vi "Begin.vi"() -> (0 "error out":errorcluster)   [LabVIEW 2013]
doc: "Called before other user functions, this VI is expected to open initial I/O refnums, load in file data, and do all program initialization. Notice that the <B>error out</B> terminal is simply used for data flow. Wiring it to other structures or subVIs ensures that this VI runs first."
uses:
  <vilib>/Rock Robotics/WPI/SafetyOutput/WPI_SafetyOutputConfigMenu.ctl
  <vilib>/Rock Robotics/WPI/DriverStation/WPI_DriverStationRobotMode2.ctl
  <vilib>/Rock Robotics/WPI/Joystick/WPI_JoystickDeviceEnum.ctl
  <vilib>/Rock Robotics/SystemInterfaces/DIO/FPGA_DIOChannel.ctl
  <vilib>/Rock Robotics/WPI/Solenoid/WPI_SolenoidChannel.ctl
  <vilib>/Rock Robotics/SystemInterfaces/DIO/FPGA_DIORelayChannel.ctl
  <vilib>/Rock Robotics/SystemInterfaces/AI/FPGA_AIChannel.ctl
  Robot Global Data.vi
  <vilib>/Rock Robotics/WPI/Counter/WPI_CounterDigitalInputToDigitalSource.vi
  <vilib>/Rock Robotics/WPI/Solenoid/WPI_SolenoidOpenSingle.vi
  <vilib>/Rock Robotics/WPI/RobotDrive/WPI_RobotDriveOpen4MotorWithCANJaguar.vi
  <vilib>/Rock Robotics/WPI/Solenoid/WPI_SolenoidOpenDouble.vi
  <vilib>/Rock Robotics/WPI/MotorControl/WPI_MotorControlOpenCANJaguar.vi
  <vilib>/Rock Robotics/WPI/Compressor/WPI_CompressorGetSetRefNum.vi
panel:
  out "error out 2":errorcluster
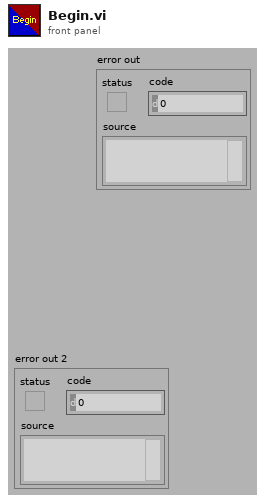
[diagram p1: front panel]
types:
  T1 = typedef "FPGA_DIOChannel.ctl" = enum8{"DIO 1", "DIO 2", "DIO 3", "DIO 4", "DIO 5", "DIO 6", "DIO 7", "DIO 8", "DIO 9", "DIO 10", "DIO 11", "DIO 12", "DIO 13", "DIO 14", "Invalid"}
  T2 = typedef "FPGA_DIORelayChannel.ctl" = enum8{"Relay 1", "Relay 2", "Relay 3", "Relay 4", "Relay 5", "Relay 6", "Relay 7", "Relay 8", "Invalid"}
  T3 = typedef "FPGA_AIChannel.ctl" = enum8{"AI 1", "AI 2", "AI 3", "AI 4", "AI 5", "AI 6", "AI 7", "AI 8", "Invalid"}
  T4 = typedef "WPI_SolenoidChannel.ctl" = enum8{"Solenoid 1", "Solenoid 2", "Solenoid 3", "Solenoid 4", "Solenoid 5", "Solenoid 6", "Solenoid 7", "Solenoid 8", "Invalid"}
  T5 = typedef "WPI_JoystickDeviceEnum.ctl" = enum16{"USB 1", "USB 2", "USB 3", "USB 4", "Kinect 1", "Kinect 2"}
  T6 = typedef "WPI_DriverStationRobotMode2.ctl" = enum16{"Autonomous Disabled", "Autonomous Enabled", "Teleop Disabled", "Teleop Enabled", "Timeout", "Finish", "Test Disabled", "Test Enabled"}
  T7 = typedef "WPI_SafetyOutputConfigMenu.ctl" = enum16{"Enable", "Disable"}
  T8 = typedef "WPI_DigitalInputDevRef.ctl" = cluster{"DevStatus":errorcluster, "DIO Channel":T1, "Digital Module":T9}
  T9 = typedef "FPGA_TypedefDigitalModule.ctl" = enum16{"Digital Module 1", "Digital Module 2"}
  T10 = typedef "FPGA_CounterEncoderSourceConvertionLVSourceType.ctl" = cluster{"DevStatus":errorcluster, "AnalogTriggerMode?":bool, "DigitalMode":cluster{"Digital Module":T9, "DIO Channel":T11}, "AnalogTriggerMode":cluster{"AnalogTriggerIndex":T12, "OutputType":T13}}
  T11 = typedef "FPGA_DIODigitalSourceChannel.ctl" = enum8{"DIO 1", "DIO 2", "DIO 3", "DIO 4", "DIO 5", "DIO 6", "DIO 7", "DIO 8", "DIO 9", "DIO 10", "DIO 11", "DIO 12", "DIO 13", "DIO 14", "Disabled"}
  T12 = typedef "FPGA_AnalogTriggerIndex.ctl" = enum8{"Trig 0", "Trig 1", "Trig 2", "Trig 3", "Trig 4", "Trig 5", "Trig 6", "Trig 7", "Invalid"}
  T13 = typedef "FPGA_AnalogTriggerOutType.ctl" = enum16{"InWindow", "TriggerState", "Rising", "Falling"}
  T14 = typedef "WPI_JoystickDevRef.ctl" = cluster{"Device":T5}
  T15 = typedef "WPI_RobotDriveDevRef.ctl" = cluster{"DevStatus":errorcluster, "Motors[]":T16[], "Square Inputs":bool, "Max Output":dbl, "Isochronous":bool}
  T16 = typedef "WPI_MotorControlDeviceRef.ctl" = cluster{"DeviceStatus":errorcluster, "Type":enum16{"PWM", "CAN"}, "PWM":cluster{"Digital Module":T9, "PWM Channel":T17, "DeadBand":T18}, "CAN":cluster{"Device Number":u8, "Control Mode":T19, "Semaphore":T20, "Max Vout":dbl}, "Invert":bool, "TransformRef":T21, "InvTransformRef":T21}
  T17 = typedef "FPGA_DIOPWMChannel.ctl" = enum8{"PWM 1", "PWM 2", "PWM 3", "PWM 4", "PWM 5", "PWM 6", "PWM 7", "PWM 8", "PWM 9", "PWM 10", "Invalid"}
  T18 = typedef "WPI_PWMDeadband.ctl" = cluster{"Name":string, "maxPositivePwm":i32, "minPositivePwm":i32, "centerPwm":i32, "maxNegativePwm":i32, "minNegativePwm":i32, "angularRange":u16}
  T19 = typedef "WPI_CANJaguar_ControlMode.ctl" = enum8{"Percent VBus", "Current", "Speed", "Position", "Voltage"}
  T20 = typedef "Semaphore RefNum" = refnum<k1>
  T21 = typedef "WPI_PWMTransform_ConPane.ctl" = refnum<vi>
  T22 = typedef "WPI_EncoderDevRef.ctl" = cluster{"DevStatus":errorcluster, "EncoderIndex":T23, "CounterIndex":T24, "DistancePerCount":dbl, "Decoding Type":T25}
  T23 = typedef "FPGA_EncoderIdx.ctl" = enum8{"Enc 0", "Enc 1", "Enc 2", "Enc 3", "Invalid"}
  T24 = typedef "FPGA_CounterCtrSystemIndex.ctl" = enum8{"Ctr 0", "Ctr 1", "Ctr 2", "Ctr 3", "Ctr 4", "Ctr 5", "Ctr 6", "Ctr 7", "Invalid"}
  T25 = typedef "WPI_EncoderType.ctl" = enum16{"1x", "2x", "4x"}
  T26 = typedef "WPI_AnalogChannelDevRef.ctl" = cluster{"DevStatus":errorcluster, "Analog Module":T27, "Analog Channel":T3}
  T27 = typedef "FPGA_TypedefAnalogModule.ctl" = enum16{"Analog Module 1", "Analog Module 2"}
  T28 = typedef "WPI_CompressorDevRef.ctl" = cluster{"DevStatus":errorcluster, "DigitalInputDevRef":T8, "RelayDevRef":T29}
  T29 = typedef "WPI_RelayDevRef.ctl" = cluster{"DevStatus":errorcluster, "Relay Channel":T2, "Digital Module":T9, "Relay Direction":T30}
  T30 = typedef "WPI_RelayDirection.ctl" = enum16{"Both directions", "Forward only", "Reverse only"}
  T31 = typedef "WPI_SolenoidDevRef.ctl" = cluster{"DevStatus":errorcluster, "Solenoid Module":T32, "Forward Solenoid Channel":T4, "Reverse Solenoid Channel":T4}
  T32 = typedef "FPGA_TypedefSolenoidModule.ctl" = enum16{"Solenoid Module 1", "Solenoid Module 2"}
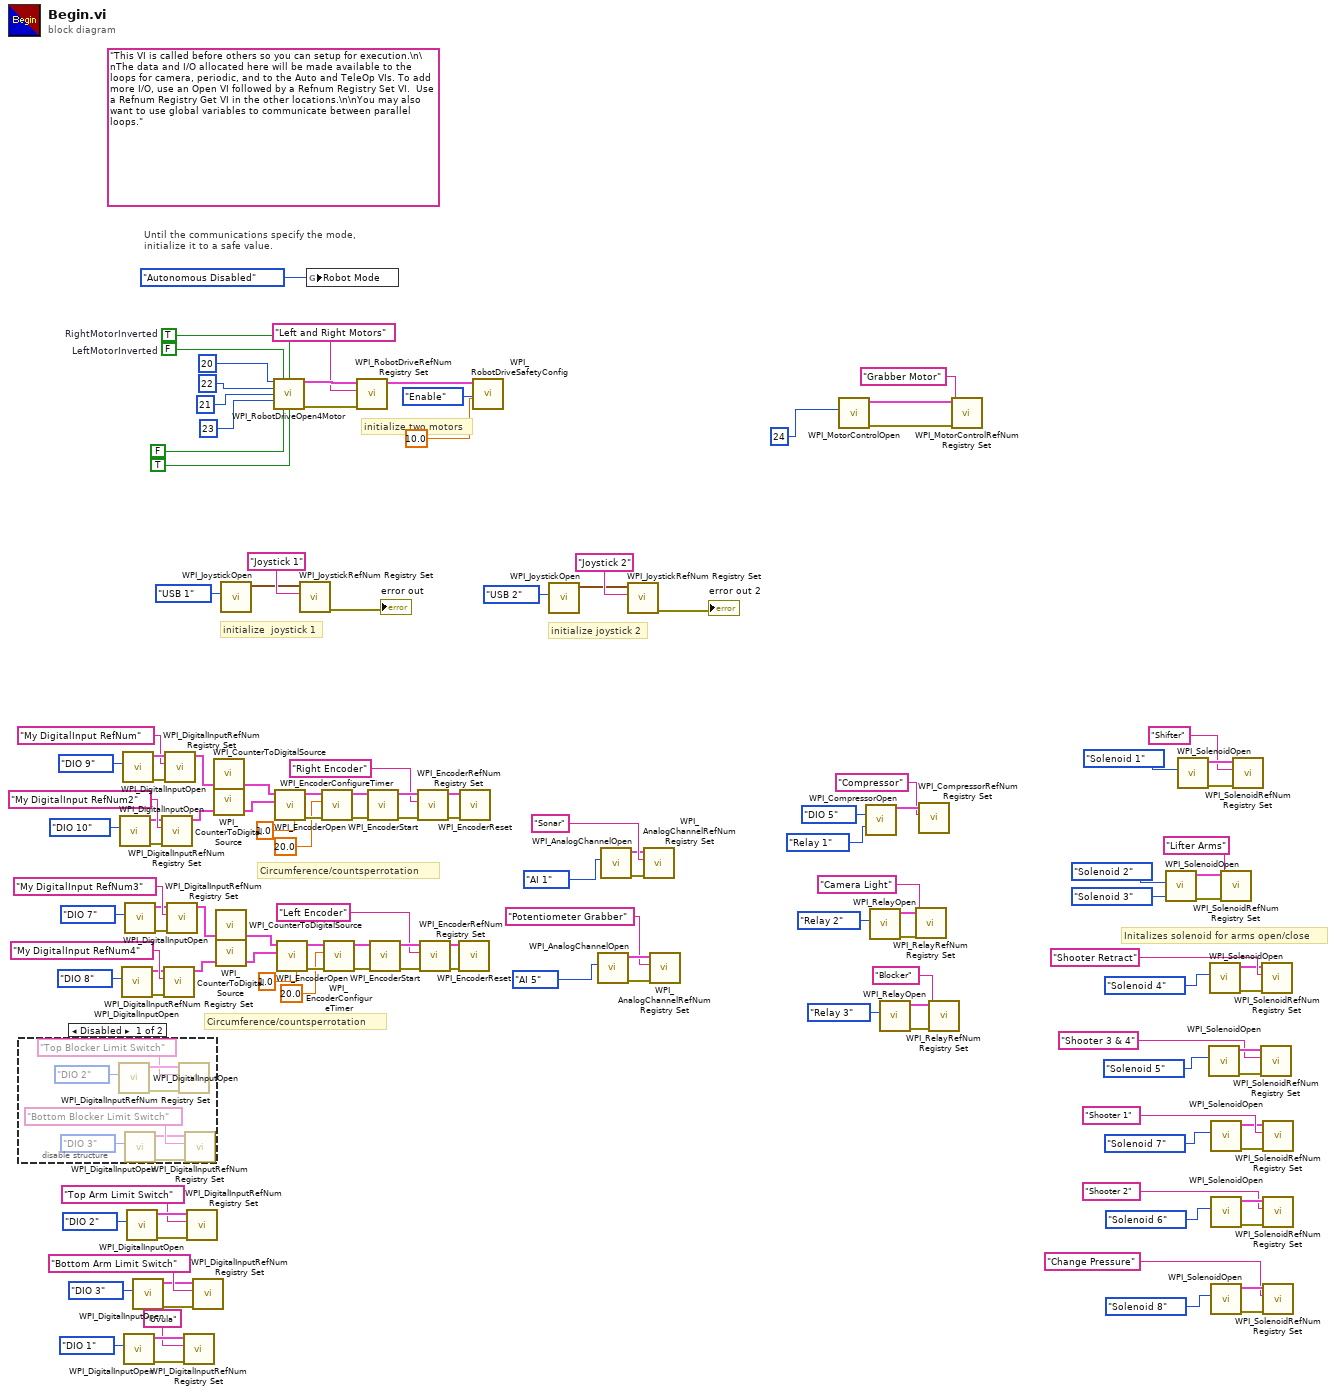
[diagram p0: block diagram]
diagram:
  (unwired) "This VI is called before others so you can setup for execution.\n\nThe data and I/O allocated here will be made available to the loops for camera, periodic, and to the Auto and TeleOp VIs. To add more I/O, use an Open VI followed by a Refnum Registry Set VI.  Use a Refnum Registry Get VI in the other locations.\n\nYou may also want to use global variables to communicate between parallel loops."
  w77 = FALSE  # LeftMotorInverted
  w76 = TRUE  # RightMotorInverted
  # "Initalizes solenoid for arms open/close"
  # "initialize joystick 2"
  # "Circumference/countsperrotation"
  # "Circumference/countsperrotation"
  # "initialize  joystick 1"
  # "Until the communications specify the mode,\ninitialize it to a safe value."
  # "initialize two motors"
  n1 = disable-structure shown="Disabled" {
    frame Disabled {
      n2 = call <vilib>:"WPI_DigitalInputOpen.vi"("DIO Channel"=FPGA_DIOChannel."DIO 2") -> ("error out"=w142:errorcluster, "DigitalInputDevRef"=w141:T8)  [unwired: 9 in]
      n3 = call <vilib>:"WPI_DigitalInputOpen.vi"("DIO Channel"=FPGA_DIOChannel."DIO 3") -> ("error out"=w135:errorcluster, "DigitalInputDevRef"=w136:T8)  [unwired: 9 in]
      n4 = call <vilib>:"WPI_DigitalInputRefNum Registry Set.vi"("error in (no error)"=w142, "refnum name"="Top Blocker Limit Switch", "DigitalInputDevRef"=w141) -> ()  [unwired: 7 in, 2 out]
      n5 = call <vilib>:"WPI_DigitalInputRefNum Registry Set.vi"("error in (no error)"=w135, "refnum name"="Bottom Blocker Limit Switch", "DigitalInputDevRef"=w136) -> ()  [unwired: 7 in, 2 out]
    }
    frame Enabled {
    }
  }
  n6 = call <vilib>:"WPI_DigitalInputOpen.vi"("DIO Channel"=FPGA_DIOChannel."DIO 10") -> ("error out"=w106:errorcluster, "DigitalInputDevRef"=w107:T8)  [unwired: 9 in]
  n7 = call <vilib>:"WPI_DigitalInputOpen.vi"("DIO Channel"=FPGA_DIOChannel."DIO 8") -> ("error out"=w101:errorcluster, "DigitalInputDevRef"=w40:T8)  [unwired: 9 in]
  n8 = call <vilib>:"WPI_DigitalInputOpen.vi"("DIO Channel"=FPGA_DIOChannel."DIO 9") -> ("error out"=w115:errorcluster, "DigitalInputDevRef"=w114:T8)  [unwired: 9 in]
  n9 = call <vilib>:"WPI_DigitalInputOpen.vi"("DIO Channel"=FPGA_DIOChannel."DIO 1") -> ("error out"=w15:errorcluster, "DigitalInputDevRef"=w14:T8)  [unwired: 9 in]
  n10 = call <vilib>:"WPI_DigitalInputOpen.vi"("DIO Channel"=FPGA_DIOChannel."DIO 7") -> ("error out"=w93:errorcluster, "DigitalInputDevRef"=w94:T8)  [unwired: 9 in]
  n11 = call <vilib>:"WPI_DigitalInputOpen.vi"("DIO Channel"=FPGA_DIOChannel."DIO 2") -> ("error out"=w27:errorcluster, "DigitalInputDevRef"=w26:T8)  [unwired: 9 in]
  n12 = call <vilib>:"WPI_DigitalInputOpen.vi"("DIO Channel"=FPGA_DIOChannel."DIO 3") -> ("error out"=w20:errorcluster, "DigitalInputDevRef"=w21:T8)  [unwired: 9 in]
  n13 = call <vilib>:"WPI_DigitalInputRefNum Registry Set.vi"("error in (no error)"=w106, "refnum name"="My DigitalInput RefNum2", "DigitalInputDevRef"=w107) -> ("DigitalInputDevRef"=w105:T8)  [unwired: 7 in, 1 out]
  n14 = call <vilib>:"WPI_DigitalInputRefNum Registry Set.vi"("error in (no error)"=w101, "refnum name"="My DigitalInput RefNum4", "DigitalInputDevRef"=w40) -> ("DigitalInputDevRef"=w102:T8)  [unwired: 7 in, 1 out]
  n15 = call <vilib>:"WPI_DigitalInputRefNum Registry Set.vi"("error in (no error)"=w115, "refnum name"="My DigitalInput RefNum", "DigitalInputDevRef"=w114) -> ("DigitalInputDevRef"=w113:T8)  [unwired: 7 in, 1 out]
  n16 = call <vilib>:"WPI_DigitalInputRefNum Registry Set.vi"("error in (no error)"=w93, "refnum name"="My DigitalInput RefNum3", "DigitalInputDevRef"=w94) -> ("DigitalInputDevRef"=w95:T8)  [unwired: 7 in, 1 out]
  n17 = call <vilib>:"WPI_DigitalInputRefNum Registry Set.vi"("error in (no error)"=w15, "refnum name"="Uvula", "DigitalInputDevRef"=w14) -> ()  [unwired: 7 in, 2 out]
  n18 = call <vilib>:"WPI_DigitalInputRefNum Registry Set.vi"("error in (no error)"=w27, "refnum name"="Top Arm Limit Switch", "DigitalInputDevRef"=w26) -> ()  [unwired: 7 in, 2 out]
  n19 = call <vilib>:"WPI_DigitalInputRefNum Registry Set.vi"("error in (no error)"=w20, "refnum name"="Bottom Arm Limit Switch", "DigitalInputDevRef"=w21) -> ()  [unwired: 7 in, 2 out]
  n20 = call-poly <vilib>:"WPI_CounterToDigitalSource.vi"("DigitalInputDevRef"=w113) -> ("Digital Source"=w116:T10)  [unwired: 6 in]
  n21 = call-poly <vilib>:"WPI_CounterToDigitalSource.vi"("DigitalInputDevRef"=w105) -> ("Digital Source"=w111:T10)  [unwired: 6 in]
  n22 = call-poly <vilib>:"WPI_CounterToDigitalSource.vi"("DigitalInputDevRef"=w95) -> ("Digital Source"=w92:T10)  [unwired: 6 in]
  n23 = call-poly <vilib>:"WPI_CounterToDigitalSource.vi"("DigitalInputDevRef"=w102) -> ("Digital Source"=w97:T10)  [unwired: 6 in]
  n24 = call <vilib>:"WPI_JoystickOpen.vi"("JoystickDevice"=WPI_JoystickDeviceEnum."USB 1") -> ("JoystickDevRef"=w128:T14)  [unwired: 10 in]
  n25 = call-poly <vilib>:"WPI_RobotDriveOpen4Motor.vi"("Rear Left Motor"=u8 20, "Rear Left Motor Inverted"=w77, "Rear Right Motor Inverted"=w76, "Rear Right Motor"=u8 22, "Front Left Motor"=u8 21, "Front Right Motor"=u8 23, "Front Left Motor Inverted"=FALSE, "Front Right Motor Inverted"=TRUE) -> ("RobotDriveDevRef"=w134:T15, "error out"=w132:errorcluster)  [unwired: 6 in]
  n26 = call <vilib>:"WPI_EncoderOpen.vi"("DistancePerCount"=1.0, "BSource"=w111, "ASource"=w116) -> ("error out"=w122:errorcluster, "EncoderDevRef"=w121:T22)  [unwired: 7 in]
  n27 = call <vilib>:"WPI_EncoderOpen.vi"("DistancePerCount"=1.0, "BSource"=w97, "ASource"=w92) -> ("error out"=w86:errorcluster, "EncoderDevRef"=w87:T22)  [unwired: 7 in]
  n28 = call <vilib>:"WPI_JoystickRefNum Registry Set.vi"("refnum name"="Joystick 1", "JoystickDevRef"=w128) -> ("error out"=→"error out":errorcluster)  [unwired: 8 in, 1 out]
  n29 = global write "Robot Global Data.vi" "Robot Mode"(WPI_DriverStationRobotMode2."Autonomous Disabled" ("Robot Mode")) -> ()
  n30 = call <vilib>:"WPI_EncoderConfigureTimer.vi"("error in (no error)"=w122, "Minimum Rate"=20.0, "EncoderDevRef"=w121) -> ("error out"=w120:errorcluster, "EncoderDevRef"=w119:T22)  [unwired: 7 in]
  n31 = call <vilib>:"WPI_EncoderConfigureTimer.vi"("error in (no error)"=w86, "Minimum Rate"=20.0, "EncoderDevRef"=w87) -> ("error out"=w88:errorcluster, "EncoderDevRef"=w89:T22)  [unwired: 7 in]
  n32 = call <vilib>:"WPI_RobotDriveRefNum Registry Set.vi"("error in (no error)"=w132, "refnum name"="Left and Right Motors", "RobotDriveDevRef"=w134) -> ("RobotDriveDevRef"=w9:T15)  [unwired: 8 out]
  n33 = call <vilib>:"WPI_EncoderStart.vi"("error in (no error)"=w120, "EncoderDevRef"=w119) -> ("error out"=w118:errorcluster, "EncoderDevRef"=w117:T22)  [unwired: 8 in]
  n34 = call <vilib>:"WPI_EncoderStart.vi"("error in (no error)"=w88, "EncoderDevRef"=w89) -> ("error out"=w90:errorcluster, "EncoderDevRef"=w91:T22)  [unwired: 8 in]
  n35 = call <vilib>:"WPI_EncoderRefNum Registry Set.vi"("error in (no error)"=w118, "refnum name"="Right Encoder", "EncoderDevRef"=w117) -> ("error out"=w2:errorcluster, "EncoderDevRef"=w1:T22)  [unwired: 7 in]
  n36 = call <vilib>:"WPI_EncoderRefNum Registry Set.vi"("error in (no error)"=w90, "refnum name"="Left Encoder", "EncoderDevRef"=w91) -> ("error out"=w4:errorcluster, "EncoderDevRef"=w3:T22)  [unwired: 7 in]
  n37 = call <vilib>:"WPI_EncoderReset.vi"("error in (no error)"=w4, "EncoderDevRef"=w3) -> ()  [unwired: 8 in, 2 out]
  n38 = call <vilib>:"WPI_EncoderReset.vi"("error in (no error)"=w2, "EncoderDevRef"=w1) -> ()  [unwired: 8 in, 2 out]
  n39 = call <vilib>:"WPI_RobotDriveSafetyConfig.vi"("timeout (s)"=10.0, "mode"=WPI_SafetyOutputConfigMenu."Enable", "RobotDriveDevRef"=w9) -> ()  [unwired: 7 in, 2 out]
  n40 = call <vilib>:"WPI_JoystickOpen.vi"("JoystickDevice"=WPI_JoystickDeviceEnum."USB 2") -> ("JoystickDevRef"=w62:T14)  [unwired: 10 in]
  n41 = call <vilib>:"WPI_AnalogChannelOpen.vi"("Analog Channel"=FPGA_AIChannel."AI 5") -> ("error out"=w59:errorcluster, "AIDeviceRef"=w58:T26)  [unwired: 9 in]
  n42 = call <vilib>:"WPI_AnalogChannelOpen.vi"("Analog Channel"=FPGA_AIChannel."AI 1") -> ("error out"=w28:errorcluster, "AIDeviceRef"=w29:T26)  [unwired: 9 in]
  n43 = call <vilib>:"WPI_JoystickRefNum Registry Set.vi"("refnum name"="Joystick 2", "JoystickDevRef"=w62) -> ("error out"=→"error out 2":errorcluster)  [unwired: 8 in, 1 out]
  n44 = call <vilib>:"WPI_AnalogChannelRefNum Registry Set.vi"("error in (no error)"=w28, "refnum name"="Sonar", "AIDeviceRef"=w29) -> ()  [unwired: 7 in, 2 out]
  n45 = call <vilib>:"WPI_AnalogChannelRefNum Registry Set.vi"("error in (no error)"=w59, "refnum name"="Potentiometer Grabber", "AIDeviceRef"=w58) -> ()  [unwired: 7 in, 2 out]
  n46 = call-poly <vilib>:"WPI_MotorControlOpen.vi"("Device Number"=u8 24) -> ("error out"=w7:errorcluster, "MotorControlDeviceRef"=w8:T16)  [unwired: 9 in]
  n47 = call <vilib>:"WPI_CompressorOpen.vi"("Pressure Switch DIO Channel"=FPGA_DIOChannel."DIO 5", "Relay Channel"=FPGA_DIORelayChannel."Relay 1") -> ("CompressorDevRef"=w65:T28)  [unwired: 12 in, 1 out]
  n48 = call <vilib>:"WPI_RelayOpen.vi"("Relay Channel"=FPGA_DIORelayChannel."Relay 2") -> ("error out"=w39:errorcluster, "RelayDevRef"=w38:T29)  [unwired: 9 in]
  n49 = call <vilib>:"WPI_RelayOpen.vi"("Relay Channel"=FPGA_DIORelayChannel."Relay 3") -> ("error out"=w19:errorcluster, "RelayDevRef"=w18:T29)  [unwired: 9 in]
  n50 = call <vilib>:"WPI_RelayRefNum Registry Set.vi"("error in (no error)"=w39, "refnum name"="Camera Light", "RelayDevRef"=w38) -> ()  [unwired: 7 in, 2 out]
  n51 = call <vilib>:"WPI_CompressorRefNum Registry Set.vi"("refnum name"="Compressor", "CompressorDevRef"=w65) -> ()  [unwired: 8 in, 2 out]
  n52 = call <vilib>:"WPI_RelayRefNum Registry Set.vi"("error in (no error)"=w19, "refnum name"="Blocker", "RelayDevRef"=w18) -> ()  [unwired: 7 in, 2 out]
  n53 = call <vilib>:"WPI_MotorControlRefNum Registry Set.vi"("error in (no error)"=w7, "refnum name"="Grabber Motor", "MotorControlDevRef"=w8) -> ()  [unwired: 7 in, 2 out]
  n54 = call-poly <vilib>:"WPI_SolenoidOpen.vi"("Reverse Solenoid Channel"=WPI_SolenoidChannel."Solenoid 3", "Forward Solenoid Channel"=WPI_SolenoidChannel."Solenoid 2") -> ("error out"=w69:errorcluster, "SolenoidDevRef"=w70:T31)  [unwired: 8 in]
  n55 = call-poly <vilib>:"WPI_SolenoidOpen.vi"("Solenoid Channel"=WPI_SolenoidChannel."Solenoid 1" ("Forward Solenoid Channel")) -> ("error out"=w81:errorcluster, "SolenoidDevRef"=w80:T31)  [unwired: 9 in]
  n56 = call-poly <vilib>:"WPI_SolenoidOpen.vi"("Solenoid Channel"=WPI_SolenoidChannel."Solenoid 5" ("Forward Solenoid Channel")) -> ("error out"=w41:errorcluster, "SolenoidDevRef"=w42:T31)  [unwired: 9 in]
  n57 = call-poly <vilib>:"WPI_SolenoidOpen.vi"("Solenoid Channel"=WPI_SolenoidChannel."Solenoid 4" ("Forward Solenoid Channel")) -> ("error out"=w32:errorcluster, "SolenoidDevRef"=w33:T31)  [unwired: 9 in]
  n58 = call-poly <vilib>:"WPI_SolenoidOpen.vi"("Solenoid Channel"=WPI_SolenoidChannel."Solenoid 7" ("Forward Solenoid Channel")) -> ("error out"=w52:errorcluster, "SolenoidDevRef"=w53:T31)  [unwired: 9 in]
  n59 = call-poly <vilib>:"WPI_SolenoidOpen.vi"("Solenoid Channel"=WPI_SolenoidChannel."Solenoid 6" ("Forward Solenoid Channel")) -> ("error out"=w47:errorcluster, "SolenoidDevRef"=w46:T31)  [unwired: 9 in]
  n60 = call-poly <vilib>:"WPI_SolenoidOpen.vi"("Solenoid Channel"=WPI_SolenoidChannel."Solenoid 8" ("Forward Solenoid Channel")) -> ("error out"=w51:errorcluster, "SolenoidDevRef"=w50:T31)  [unwired: 9 in]
  n61 = call <vilib>:"WPI_SolenoidRefNum Registry Set.vi"("error in (no error)"=w69, "refnum name"="Lifter Arms", "SolenoidDevRef"=w70) -> ()  [unwired: 7 in, 2 out]
  n62 = call <vilib>:"WPI_SolenoidRefNum Registry Set.vi"("error in (no error)"=w81, "refnum name"="Shifter", "SolenoidDevRef"=w80) -> ()  [unwired: 7 in, 2 out]
  n63 = call <vilib>:"WPI_SolenoidRefNum Registry Set.vi"("error in (no error)"=w41, "refnum name"="Shooter 3 & 4", "SolenoidDevRef"=w42) -> ()  [unwired: 7 in, 2 out]
  n64 = call <vilib>:"WPI_SolenoidRefNum Registry Set.vi"("error in (no error)"=w32, "refnum name"="Shooter Retract", "SolenoidDevRef"=w33) -> ()  [unwired: 7 in, 2 out]
  n65 = call <vilib>:"WPI_SolenoidRefNum Registry Set.vi"("error in (no error)"=w52, "refnum name"="Shooter 1", "SolenoidDevRef"=w53) -> ()  [unwired: 7 in, 2 out]
  n66 = call <vilib>:"WPI_SolenoidRefNum Registry Set.vi"("error in (no error)"=w47, "refnum name"="Shooter 2", "SolenoidDevRef"=w46) -> ()  [unwired: 7 in, 2 out]
  n67 = call <vilib>:"WPI_SolenoidRefNum Registry Set.vi"("error in (no error)"=w51, "refnum name"="Change Pressure", "SolenoidDevRef"=w50) -> ()  [unwired: 7 in, 2 out]
